vi "CaculateStringControl.vi"(10 "stringControl":refnum<vi> caption="컨트롤 참조 번호", 11 "category":enum16{"add", "minus"}(ring)) -> ()   [LabVIEW 2018]
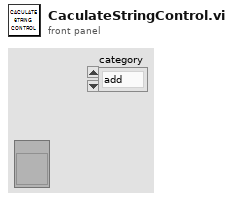
[diagram p1: front panel]
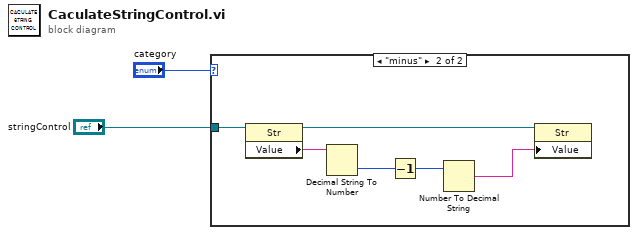
[diagram p0: block diagram]
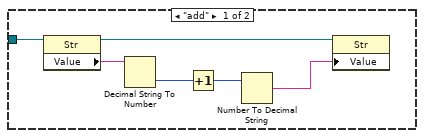
[diagram p2: hidden frame]
diagram:
  n1 = case shown="\"minus\"" "category" {
    tunnel: "stringControl" -> [w8 w14]
    frame "add" {
      n2 = property class="Str"(reference=w8) -> (reference out=w6:refnum<vi>, "Value"=w7:string)  [unwired: 1 in, 1 out]
      n3 = Decimal String To Number(string=w7) -> (number=w5:i32)  [unwired: 2 in, 1 out]
      n4 = Increment(x=w5) -> (x+1=w4:i32)
      n5 = Number To Decimal String(number=w4) -> (decimal integer string=w3:string)  [unwired: 1 in]
      n6 = property class="Str"(reference=w6, "Value"=w3) -> ()  [unwired: 1 in, 2 out]
    }
    frame "minus" {
      n7 = property class="Str"(reference=w14) -> (reference out=w12:refnum<vi>, "Value"=w13:string)  [unwired: 1 in, 1 out]
      n8 = Decimal String To Number(string=w13) -> (number=w11:i32)  [unwired: 2 in, 1 out]
      n9 = Decrement(x=w11) -> (x-1=w10:i32)
      n10 = Number To Decimal String(number=w10) -> (decimal integer string=w9:string)  [unwired: 1 in]
      n11 = property class="Str"(reference=w12, "Value"=w9) -> ()  [unwired: 1 in, 2 out]
    }
  }
